vi "Read VISAHandle.vi"(8 "error in (no error)":errorcluster, 11 "Keysight335XX in":refnum<class "Keysight335XX.lvclass">) -> (0 "error out":errorcluster, 2 "VISAHandle":refnum<visa-resource-name>, 3 "Keysight335XX out":refnum<class "Keysight335XX.lvclass">)   [LabVIEW 2014, in "FGenPlugins.lvlib" / "Keysight335XX.lvclass"]
uses:
  Keysight335XX.lvclass
  Keysight335XX.lvclass/Keysight335XX.ctl
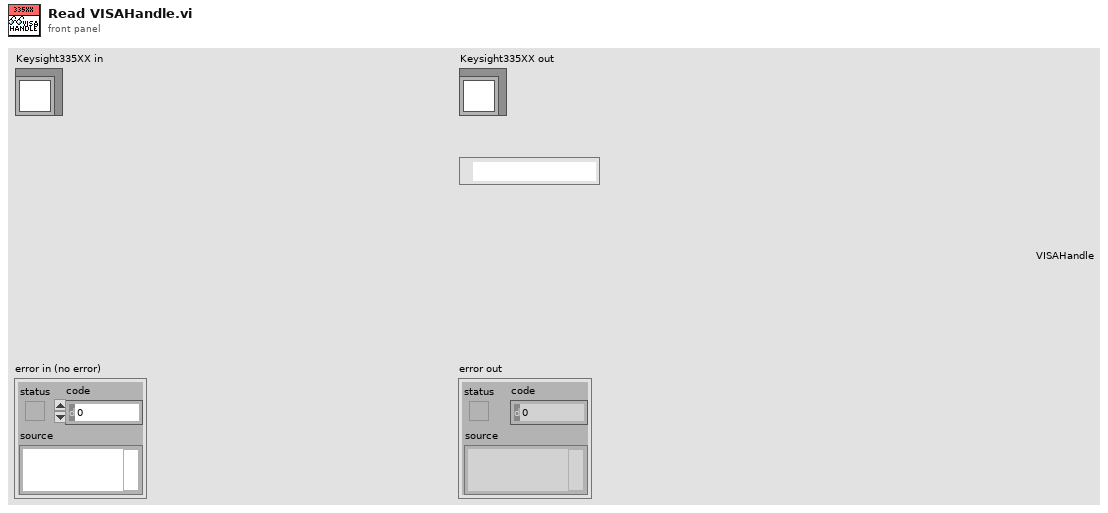
[diagram p1: front panel]
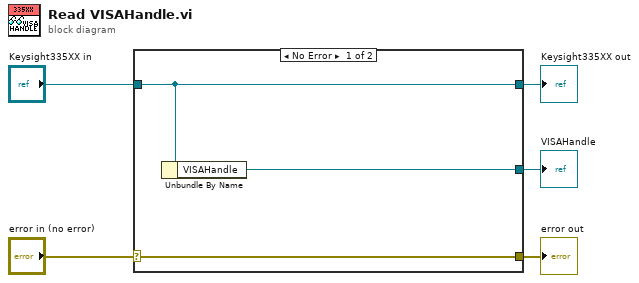
[diagram p0: block diagram]
diagram:
  n1 = case shown="No Error" "error in (no error)" {
    selector: "error in (no error)" -> [w8 w9]
    tunnel: [w8 w9] -> w4
    tunnel: [w7 w10] -> w2
    tunnel: "Keysight335XX in" -> [w7 w10]
    tunnel: [w6 _] -> w1
    frame No Error {
      n2 = Unbundle By Name(w7) -> ("VISAHandle"=w6:refnum<visa-resource-name>)
    }
    frame Error {
    }
  }
  "error out" <- w4
  "Keysight335XX out" <- w2
  "VISAHandle" <- w1
